vi "JAUS SimpleServices.vi"() -> ()   [LabVIEW 2009]
uses:
  Support Files/JUDP Write Queue Element.ctl
  Support Files/Simple Services Receive Triggers.ctl
  Support Files/Address.ctl
  Support Files/ServiceRec.ctl
panel:
  out "Velocity State Sensor Added?":bool
  out "Discovery Added?":bool
  out "JAUS Loop":bool
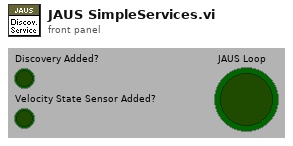
[diagram p1: front panel]
types:
  T1 = typedef "Simple Services Receive Triggers.ctl" = enum16{"NULL", "ReceiveQueryIdentification", "ReceiveQueryServices", "ReceiveQueryVelocityState"}
  T2 = typedef "Address.ctl" = cluster{"Subsystem Id":u16, "Node Id":u8, "Component Id":u8}
  T3 = cluster{"Trigger":T1, "Payload":string, "Sender ID":T2}
  T4 = typedef "JUDP Write Queue Element.ctl" = cluster{"Encoded JAUS Message":string, "Destination ID":u32}
  T5 = typedef "ServiceRec.ctl" = cluster{"ServiceURI":string, "MajorVerNum":u8, "MinorVerNum":u8}
  T6 = typedef "NodeRec.ctl" = cluster{"Node Id":u8, "ComponentSeq":T7[]}
  T7 = typedef "ComponentRec.ctl" = cluster{"Component Id":u8, "Instance Id":u8, "ServiceSeq":T5[]}
  T8 = typedef "VelocityState.ctl" = cluster{"Velocity X":dbl, "Velocity Y":dbl, "Velocity Z":dbl, "Velocity RMS":dbl, "Roll Rate":dbl, "Pitch Rate":dbl, "Yaw Rate":dbl, "Rate RMS":dbl, "TimeRec":T9}
  T9 = typedef "TimeRec.ctl" = cluster{"Milliseconds":u32, "Seconds":u32, "Minutes":u32, "Hours":u32, "Day":u32}
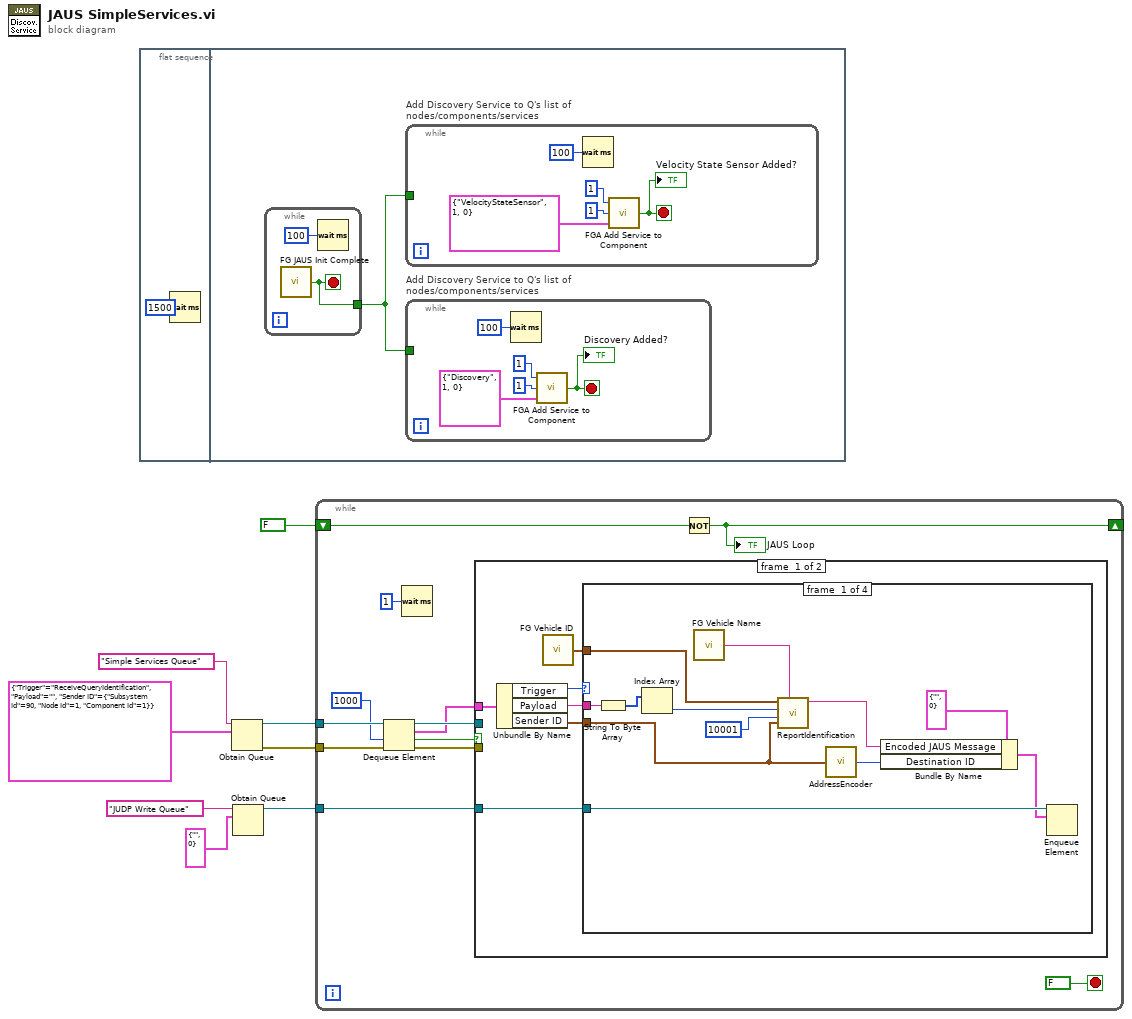
[diagram p0: block diagram]
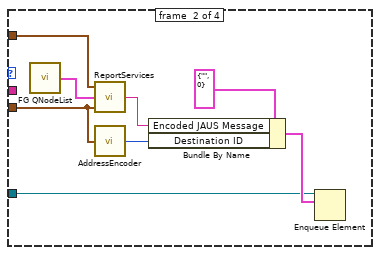
[diagram p2: hidden frame]
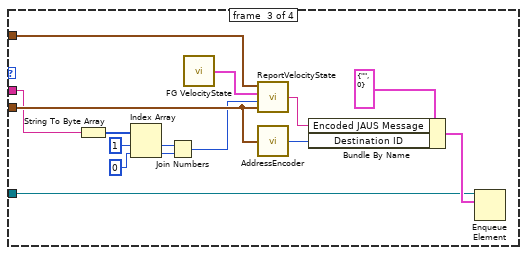
[diagram p3: hidden frame]
diagram:
  n1 = flat-sequence {
    frame #0 {
      n2 = Wait (ms)(milliseconds to wait=u32 1500) -> ()  [unwired: 1 out]
    }
    frame #1 {
      n3 = while "sdvsd" {
        tunnel: [w21] -> w10
        stop <- w21 stop-if-true
        n4 = call "FG JAUS Init Complete.vi"() -> ("Init Complete out"=w21:bool)  [unwired: 2 in]
        n5 = Wait (ms)(milliseconds to wait=u32 100) -> ()  [unwired: 1 out]
      }
      n6 = while "Add Discovery Service to Q's list of \nnodes/components/services" {
        tunnel: w10 -> [_]
        stop <- w12 stop-if-true
        n7 = Wait (ms)(milliseconds to wait=u32 100) -> ()  [unwired: 1 out]
        n8 = call "FGA Add Service to Component.vi"("ServiceRec"=T5 {"ServiceURI"="VelocityStateSensor", "MajorVerNum"=1, "MinorVerNum"=0}, "Component Id"=u8 1, "Node Id"=u8 1) -> ("Added?"=w12:bool)
        "Velocity State Sensor Added?" <- w12
      }
      n9 = while "Add Discovery Service to Q's list of \nnodes/components/services" {
        tunnel: w10 -> [_]
        stop <- w17 stop-if-true
        n10 = Wait (ms)(milliseconds to wait=u32 100) -> ()  [unwired: 1 out]
        n11 = call "FGA Add Service to Component.vi"("ServiceRec"=T5 {"ServiceURI"="Discovery", "MajorVerNum"=1, "MinorVerNum"=0}, "Component Id"=u8 1, "Node Id"=u8 1) -> ("Added?"=w17:bool)
        "Discovery Added?" <- w17
      }
    }
  }
  n12 = Obtain Queue(name (unnamed)="Simple Services Queue", element data type=T3 {"Trigger"=enum."ReceiveQueryIdentification", "Payload"="", "Sender ID"={"Subsystem Id"=90, "Node Id"=1, "Component Id"=1}} ("Receive FSM Queue Element")) -> (queue out=w7:refnum<queue>, error out=w8:errorcluster)  [unwired: 3 in, 1 out]
  n13 = Obtain Queue(name (unnamed)="JUDP Write Queue", element data type=T4 {"Encoded JAUS Message"="", "Destination ID"=0} ("Cluster")) -> (queue out=w5:refnum<queue>)  [unwired: 3 in, 2 out]
  n14 = while {
    tunnel: w7 -> [w34]
    tunnel: w8 -> [w33]
    shift-right: [w27] -> _
    shift-left: FALSE ("stop") -> [w26]
    tunnel: w5 -> [w25]
    stop <- FALSE stop-if-true
    n15 = Dequeue Element(queue=w34, timeout in ms (-1)=1000, error in (no error)=w33) -> (queue out=w30:refnum<queue>, element=w28:T3, timed out?=w31:bool, error out=w29:errorcluster)
    n16 = Wait (ms)(milliseconds to wait=u32 1) -> ()  [unwired: 1 out]
    n17 = case shown="False" w31 {
      tunnel: w30 -> [_ _]
      tunnel: w29 -> [_ _]
      tunnel: w28 -> [w40 _]
      tunnel: w25 -> [w36 _]
      frame #0 {
        n18 = Unbundle By Name(w40) -> ("Trigger"=w39:T1, "Payload"=w38:string, "Sender ID"=w37:T2)
        n19 = call "FG Vehicle ID.vi"() -> ("Vehicle ID out"=w35:T2)  [unwired: 2 in]
        n20 = case shown="\"ReceiveQueryIdentification\", Default" w39 {
          tunnel: w38 -> [w52 _ w68 _]
          tunnel: w37 -> [w43 w58 w69 _]
          tunnel: w36 -> [w48 w54 w71 _]
          tunnel: w35 -> [w41 w56 w70 _]
          frame #0 {
            n21 = String To Byte Array(string=w52) -> (unsigned byte array=w51:u8[])
            n22 = Index Array(array=w51) -> (element=w50:u8)  [unwired: 1 in]
            n23 = call "FG Vehicle Name.vi"() -> ("Vehicle Name out"=w42:string)  [unwired: 2 in]
            n24 = call "ReportIdentification.vi"("Vehicle Name"=w42, "Destination"=w43, "Type"=u16 10001, "QueryType"=w50, "Source"=w41) -> ("Encoded JAUS Message"=w46:string)  [unwired: 6 in]
            n25 = call "AddressEncoder.vi"("Address Cluster"=w43) -> ("Address"=w47:u32)
            n26 = Bundle By Name(cluster=T4 {"Encoded JAUS Message"="", "Destination ID"=0} ("Cluster"), "Encoded JAUS Message"=w46, "Destination ID"=w47) -> (w44:T4)
            n27 = Enqueue Element(queue=w48, element=w44) -> ()  [unwired: 2 in, 3 out]
          }
          frame #1 {
            n28 = call "FG QNodeList.vi"() -> ("NodeList out"=w53:T6[])  [unwired: 2 in]
            n29 = call "ReportServices.vi"("Destination"=w58, "NodeList"=w53, "Source"=w56) -> ("Encoded JAUS Message"=w55:string)
            n30 = call "AddressEncoder.vi"("Address Cluster"=w58) -> ("Address"=w57:u32)
            n31 = Bundle By Name(cluster=T4 {"Encoded JAUS Message"="", "Destination ID"=0} ("Cluster"), "Encoded JAUS Message"=w55, "Destination ID"=w57) -> (w59:T4)
            n32 = Enqueue Element(queue=w54, element=w59) -> ()  [unwired: 2 in, 3 out]
          }
          frame #2 {
            n33 = String To Byte Array(string=w68) -> (unsigned byte array=w67:u8[])
            n34 = Index Array(array=w67, index #1=1 ("index"), index #2=0 ("index")) -> (element #1=w64:u8, element #2=w63:u8)
            n35 = Join Numbers(hi=w64, lo=w63) -> ((hi.lo)=w62:u16)
            n36 = call "FG VelocityState.vi"() -> ("VelocityState out"=w61:T8)  [unwired: 2 in]
            n37 = call "ReportVelocityState.vi"("Destination"=w69, "PresenceVector"=w62, "VelocityState"=w61, "Source"=w70) -> ("Encoded JAUS Message"=w72:string)
            n38 = call "AddressEncoder.vi"("Address Cluster"=w69) -> ("Address"=w73:u32)
            n39 = Bundle By Name(cluster=T4 {"Encoded JAUS Message"="", "Destination ID"=0} ("Cluster"), "Encoded JAUS Message"=w72, "Destination ID"=w73) -> (w74:T4)
            n40 = Enqueue Element(queue=w71, element=w74) -> ()  [unwired: 2 in, 3 out]
          }
          frame #3 {
          }
        }
      }
      frame #1 {
      }
    }
    n41 = Not(x=w26) -> (.not. x?=w27:bool)
    "JAUS Loop" <- w27
  }
